vi "AC Transport Measure.vi"(0 "SR860 Ch1 Address":string="4", 1 "Ch1 Enable":bool=TRUE, 2 "Buffer Offset (kb)":string="0", 3 "Buffer Size (kb)":i32=2, 4 "Ch2 Enable":bool, 5 "SR860 Ch2 Address":string="5") -> (12 "R1 Mean":dbl=3.2285320727964972e-06, 13 "R2 Mean":dbl=2.497260236822285e-05, 14 "R1 STD":dbl=8.930686760684023e-10, 15 "T1 Mean":dbl=2.6491355067119002, 16 "T1 STD":dbl=0.013498646334936281, 17 "T2 STD":dbl=2.4806903153139386, 18 "T2 Mean":dbl=-15.289178885519505, 19 "R2 STD":dbl=2.0281499748667416e-06)   [LabVIEW 2020]
uses:
  <vilib>/Analysis/NI_AALBase.lvlib
panel:
  out "Sign2":i8
  out "Garbage 1":string
  out "Sign1":i8
  in  "Sign Correction":bool=TRUE
  out "Garbage Buffer 2":errorcluster
  out "Garbage 2":string
  out "n":i32
  out "number of bytes":i32
  out "cccc":string
  out "#n":string
  out "Garbage Buffer 1":errorcluster
  in  "Measure New?":bool=TRUE
  out "Error SR860 Ch1 2":errorcluster
  out "Buffer 2":sgl[](array[numeric])=[2.0345116e-05, -18.978868, 2.0385167e-05, -18.834179, 2.042573e-05, -18.690664, 2.0466812e-05, -18.548409, 2.0508425e-05, -18.407497, 2.0550568e-05, -18.26797, 2.0593256e-05, -18.129843, 2.0636486e-05, -17.993101, 2.0680263e-05, -17.857708, 2.0724583e-05, -17.723639, 2.0769432e-05, -17.59087, 2.0814796e-05, -17.459414, 2.0860638e-05, -17.32928, 2.0906931e-05, -17.200508, 2.0953643e-05, -17.07314, 2.1000751e-05, -16.947222, 2.1048243e-05, -16.822803, 2.1096113e-05, -16.699953, 2.1144375e-05, -16.578714, 2.1193024e-05, -16.459133, 2.1242071e-05, -16.341232, 2.1291504e-05, -16.224995, 2.134132e-05, -16.110392, 2.1391503e-05, -15.997362, 2.1442036e-05, -15.885857, 2.1492897e-05, -15.775839, 2.1544056e-05, -15.667302, 2.1595477e-05, -15.560262, 2.1647133e-05, -15.454752, 2.1698983e-05, -15.35082, 2.1750997e-05, -15.248506, 2.1803164e-05, -15.147846, 2.1855478e-05, -15.048877, 2.1907945e-05, -14.951616, 2.196056e-05, -14.856077, 2.2013332e-05, -14.762263, 2.2066246e-05, -14.670146, 2.2119291e-05, -14.579687, 2.2172442e-05, -14.490837, 2.2225673e-05, -14.403539, 2.2278957e-05, -14.317757, 2.2332262e-05, -14.233484, 2.238556e-05, -14.150742, 2.243882e-05, -14.069578, 2.2492019e-05, -13.990051, 2.2545135e-05, -13.912204, 2.2598155e-05, -13.836069, 2.2651084e-05, -13.761671, 2.2703925e-05, -13.6890135, 2.2756687e-05, -13.618082, 2.2809376e-05, -13.548866, 2.2861985e-05, -13.481344, 2.2914506e-05, -13.415473, 2.2966908e-05, -13.351213, 2.3019165e-05, -13.288529, 2.307125e-05, -13.22739, 2.312314e-05, -13.167805, 2.317481e-05, -13.109787, 2.3226246e-05, -13.053399, 2.3277438e-05, -12.998701, 2.3328375e-05, -12.945737, 2.3379056e-05, -12.894549, 2.3429491e-05, -12.845147, 2.3479688e-05, -12.797515, 2.3529663e-05, -12.751628, 2.3579429e-05, -12.707447, 2.3628983e-05, -12.664949, 2.3678318e-05, -12.624104, 2.3727416e-05, -12.584871, 2.3776249e-05, -12.547233, 2.3824798e-05, -12.511176, 2.3873035e-05, -12.476706, 2.3920955e-05, -12.44384, 2.3968558e-05, -12.41263, 2.4015842e-05, -12.383121, 2.4062814e-05, -12.355357, 2.4109488e-05, -12.329361, 2.4155874e-05, -12.305133, 2.4201987e-05, -12.282635, 2.4247842e-05, -12.261823, 2.4293442e-05, -12.242645, 2.4338806e-05, -12.225046, 2.4383913e-05, -12.208999, 2.4428757e-05, -12.194475, 2.447331e-05, -12.18147, 2.4517547e-05, -12.169972, 2.456146e-05, -12.159997, 2.4605035e-05, -12.151553, 2.4648285e-05, -12.144676, 2.4691219e-05, -12.139395, 2.4733852e-05, -12.135744, 2.4776204e-05, -12.133726, 2.4818284e-05, -12.133321, 2.4860108e-05, -12.134499, 2.4901683e-05, -12.137181, 2.4943007e-05, -12.141312, 2.4984087e-05, -12.1468315, 2.502491e-05, -12.153699, 2.5065463e-05, -12.161902, 2.5105717e-05, -12.1714325, 2.514566e-05, -12.182309, 2.518527e-05, -12.194537, 2.5224552e-05, -12.20814, 2.5263502e-05, -12.223128, 2.5302144e-05, -12.239519, 2.534049e-05, -12.257316, 2.5378566e-05, -12.276516, 2.5416373e-05, -12.297089, 2.545392e-05, -12.318993, 2.5491205e-05, -12.342162, 2.552821e-05, -12.366525, 2.5564932e-05, -12.392026, 2.5601348e-05, -12.418632, 2.5637439e-05, -12.446331, 2.5673184e-05, -12.475138, 2.570856e-05, -12.505072, 2.574355e-05, -12.536165, 2.577815e-05, -12.568429, 2.5812364e-05, -12.601876, 2.58462e-05, -12.636499, 2.587968e-05, -12.672294, 2.5912816e-05, -12.709234, 2.5945612e-05, -12.747284, 2.5978066e-05, -12.786409, 2.6010159e-05, -12.826544, 2.6041876e-05, -12.867631, 2.607319e-05, -12.90963, 2.6104071e-05, -12.952507, 2.6134505e-05, -12.996262, 2.616447e-05, -13.040911, 2.6193942e-05, -13.086489, 2.622292e-05, -13.133036, 2.6251388e-05, -13.18057, 2.6279351e-05, -13.22909, 2.630681e-05, -13.27858, 2.633379e-05, -13.329011, 2.636029e-05, -13.380347, 2.638632e-05, -13.432542, 2.641187e-05, -13.485546, 2.6436916e-05, -13.539323, 2.6461428e-05, -13.593819, 2.6485382e-05, -13.649003, 2.6508755e-05, -13.704853, 2.6531518e-05, -13.761367, 2.6553664e-05, -13.818572, 2.6575182e-05, -13.876489, 2.6596077e-05, -13.935158, 2.6616346e-05, -13.994596, 2.6635995e-05, -14.054795, 2.6655029e-05, -14.115723, 2.6673462e-05, -14.177329, 2.6691305e-05, -14.239562, 2.6708554e-05, -14.302363, 2.6725202e-05, -14.365683, 2.6741236e-05, -14.429477, 2.6756623e-05, -14.493724, 2.6771333e-05, -14.558396, 2.6785352e-05, -14.62348, 2.6798662e-05, -14.688981, 2.681126e-05, -14.754904, 2.6823154e-05, -14.821272, 2.6834356e-05, -14.888111, 2.6844878e-05, -14.9554205, 2.6854741e-05, -15.023187, 2.6863952e-05, -15.091367, 2.6872523e-05, -15.1599045, 2.6880463e-05, -15.2287245, 2.6887777e-05, -15.297751, 2.6894459e-05, -15.366936, 2.6900496e-05, -15.43625, 2.6905873e-05, -15.505663, 2.6910573e-05, -15.5751705, 2.6914571e-05, -15.644768, 2.6917876e-05, -15.714455, 2.692049e-05, -15.784235, 2.6922431e-05, -15.854111, 2.6923728e-05, -15.924088, 2.6924405e-05, -15.994141, 2.6924477e-05, -16.064253, 2.6923977e-05, -16.134369, 2.6922904e-05, -16.204422, 2.6921272e-05, -16.274336, 2.6919075e-05, -16.34403, 2.691632e-05, -16.413458, 2.6912998e-05, -16.482584, 2.6909103e-05, -16.551395, 2.690463e-05, -16.6199, 2.6899572e-05, -16.688105, 2.6893942e-05, -16.756018, 2.688775e-05, -16.823635, 2.6881024e-05, -16.89094, 2.6873802e-05, -16.957922, 2.6866119e-05, -17.02454, 2.6857995e-05, -17.090763, 2.6849453e-05, -17.156532, 2.6840504e-05, -17.221783, 2.683114e-05, -17.286438, 2.6821364e-05, -17.35044, 2.6811176e-05, -17.413725, 2.6800566e-05, -17.476278, 2.6789536e-05, -17.538095, 2.6778089e-05, -17.599197, 2.6766227e-05, -17.659603, 2.6753964e-05, -17.719322, 2.6741316e-05, -17.77836, 2.6728316e-05, -17.83669, 2.6714988e-05, -17.89429, 2.6701373e-05, -17.951107, 2.6687494e-05, -18.007095, 2.6673364e-05, -18.062208, 2.6658987e-05, -18.116385, 2.6644357e-05, -18.169582, 2.6629465e-05, -18.221745, 2.6614305e-05, -18.27284, 2.6598864e-05, -18.322859, 2.658315e-05, -18.371809, 2.656717e-05, -18.419716, 2.6550935e-05, -18.466608, 2.6534459e-05, -18.512505, 2.6517757e-05, -18.557413, 2.6500858e-05, -18.601297, 2.6483782e-05, -18.644125, 2.646656e-05, -18.685831, 2.64492e-05, -18.726366, 2.6431719e-05, -18.765667, 2.6414105e-05, -18.803701, 2.6396354e-05, -18.84043, 2.6378446e-05, -18.875816, 2.6360369e-05, -18.90985, 2.6342113e-05, -18.942524, 2.6323685e-05, -18.973843, 2.6305092e-05, -19.003841, 2.6286354e-05, -19.032534, 2.6267498e-05, -19.059935, 2.6248541e-05, -19.08605, 2.62295e-05, -19.110842, 2.6210393e-05, -19.13426, 2.6191248e-05, -19.156242, 2.617207e-05, -19.176723, 2.6152864e-05, -19.195648, 2.6133623e-05, -19.212978, 2.6114341e-05, -19.228697, 2.6095006e-05, -19.242796, 2.6075599e-05, -19.255272, 2.6056116e-05, -19.26614, 2.6036569e-05, -19.275402, 2.6016975e-05, -19.28308, 2.5997351e-05, -19.289183, 2.5977739e-05, -19.29372, 2.5958156e-05, -19.296686, 2.5938614e-05, -19.298044, 2.5919142e-05, -19.297743, 2.589974e-05, -19.295721, 2.588042e-05, -19.291908, 2.5861173e-05, -19.286263, 2.5842002e-05, -19.278759]
  out "Buffer 2":string
  out "size(s) 2":i32=512
  out "R2 Buffer":sgl[](array[numeric])=[2.0345116e-05, 2.0385167e-05, 2.042573e-05, 2.0466812e-05, 2.0508425e-05, 2.0550568e-05, 2.0593256e-05, 2.0636486e-05, 2.0680263e-05, 2.0724583e-05, 2.0769432e-05, 2.0814796e-05, 2.0860638e-05, 2.0906931e-05, 2.0953643e-05, 2.1000751e-05, 2.1048243e-05, 2.1096113e-05, 2.1144375e-05, 2.1193024e-05, 2.1242071e-05, 2.1291504e-05, 2.134132e-05, 2.1391503e-05, 2.1442036e-05, 2.1492897e-05, 2.1544056e-05, 2.1595477e-05, 2.1647133e-05, 2.1698983e-05, 2.1750997e-05, 2.1803164e-05, 2.1855478e-05, 2.1907945e-05, 2.196056e-05, 2.2013332e-05, 2.2066246e-05, 2.2119291e-05, 2.2172442e-05, 2.2225673e-05, 2.2278957e-05, 2.2332262e-05, 2.238556e-05, 2.243882e-05, 2.2492019e-05, 2.2545135e-05, 2.2598155e-05, 2.2651084e-05, 2.2703925e-05, 2.2756687e-05, 2.2809376e-05, 2.2861985e-05, 2.2914506e-05, 2.2966908e-05, 2.3019165e-05, 2.307125e-05, 2.312314e-05, 2.317481e-05, 2.3226246e-05, 2.3277438e-05, 2.3328375e-05, 2.3379056e-05, 2.3429491e-05, 2.3479688e-05, 2.3529663e-05, 2.3579429e-05, 2.3628983e-05, 2.3678318e-05, 2.3727416e-05, 2.3776249e-05, 2.3824798e-05, 2.3873035e-05, 2.3920955e-05, 2.3968558e-05, 2.4015842e-05, 2.4062814e-05, 2.4109488e-05, 2.4155874e-05, 2.4201987e-05, 2.4247842e-05, 2.4293442e-05, 2.4338806e-05, 2.4383913e-05, 2.4428757e-05, 2.447331e-05, 2.4517547e-05, 2.456146e-05, 2.4605035e-05, 2.4648285e-05, 2.4691219e-05, 2.4733852e-05, 2.4776204e-05, 2.4818284e-05, 2.4860108e-05, 2.4901683e-05, 2.4943007e-05, 2.4984087e-05, 2.502491e-05, 2.5065463e-05, 2.5105717e-05, 2.514566e-05, 2.518527e-05, 2.5224552e-05, 2.5263502e-05, 2.5302144e-05, 2.534049e-05, 2.5378566e-05, 2.5416373e-05, 2.545392e-05, 2.5491205e-05, 2.552821e-05, 2.5564932e-05, 2.5601348e-05, 2.5637439e-05, 2.5673184e-05, 2.570856e-05, 2.574355e-05, 2.577815e-05, 2.5812364e-05, 2.58462e-05, 2.587968e-05, 2.5912816e-05, 2.5945612e-05, 2.5978066e-05, 2.6010159e-05, 2.6041876e-05, 2.607319e-05, 2.6104071e-05, 2.6134505e-05, 2.616447e-05, 2.6193942e-05, 2.622292e-05, 2.6251388e-05, 2.6279351e-05, 2.630681e-05, 2.633379e-05, 2.636029e-05, 2.638632e-05, 2.641187e-05, 2.6436916e-05, 2.6461428e-05, 2.6485382e-05, 2.6508755e-05, 2.6531518e-05, 2.6553664e-05, 2.6575182e-05, 2.6596077e-05, 2.6616346e-05, 2.6635995e-05, 2.6655029e-05, 2.6673462e-05, 2.6691305e-05, 2.6708554e-05, 2.6725202e-05, 2.6741236e-05, 2.6756623e-05, 2.6771333e-05, 2.6785352e-05, 2.6798662e-05, 2.681126e-05, 2.6823154e-05, 2.6834356e-05, 2.6844878e-05, 2.6854741e-05, 2.6863952e-05, 2.6872523e-05, 2.6880463e-05, 2.6887777e-05, 2.6894459e-05, 2.6900496e-05, 2.6905873e-05, 2.6910573e-05, 2.6914571e-05, 2.6917876e-05, 2.692049e-05, 2.6922431e-05, 2.6923728e-05, 2.6924405e-05, 2.6924477e-05, 2.6923977e-05, 2.6922904e-05, 2.6921272e-05, 2.6919075e-05, 2.691632e-05, 2.6912998e-05, 2.6909103e-05, 2.690463e-05, 2.6899572e-05, 2.6893942e-05, 2.688775e-05, 2.6881024e-05, 2.6873802e-05, 2.6866119e-05, 2.6857995e-05, 2.6849453e-05, 2.6840504e-05, 2.683114e-05, 2.6821364e-05, 2.6811176e-05, 2.6800566e-05, 2.6789536e-05, 2.6778089e-05, 2.6766227e-05, 2.6753964e-05, 2.6741316e-05, 2.6728316e-05, 2.6714988e-05, 2.6701373e-05, 2.6687494e-05, 2.6673364e-05, 2.6658987e-05, 2.6644357e-05, 2.6629465e-05, 2.6614305e-05, 2.6598864e-05, 2.658315e-05, 2.656717e-05, 2.6550935e-05, 2.6534459e-05, 2.6517757e-05, 2.6500858e-05, 2.6483782e-05, 2.646656e-05, 2.64492e-05, 2.6431719e-05, 2.6414105e-05, 2.6396354e-05, 2.6378446e-05, 2.6360369e-05, 2.6342113e-05, 2.6323685e-05, 2.6305092e-05, 2.6286354e-05, 2.6267498e-05, 2.6248541e-05, 2.62295e-05, 2.6210393e-05, 2.6191248e-05, 2.617207e-05, 2.6152864e-05, 2.6133623e-05, 2.6114341e-05, 2.6095006e-05, 2.6075599e-05, 2.6056116e-05, 2.6036569e-05, 2.6016975e-05, 2.5997351e-05, 2.5977739e-05, 2.5958156e-05, 2.5938614e-05, 2.5919142e-05, 2.589974e-05, 2.588042e-05, 2.5861173e-05, 2.5842002e-05]
  out "T2 Buffer":sgl[](array[numeric])=[-18.978868, -18.834179, -18.690664, -18.548409, -18.407497, -18.26797, -18.129843, -17.993101, -17.857708, -17.723639, -17.59087, -17.459414, -17.32928, -17.200508, -17.07314, -16.947222, -16.822803, -16.699953, -16.578714, -16.459133, -16.341232, -16.224995, -16.110392, -15.997362, -15.885857, -15.775839, -15.667302, -15.560262, -15.454752, -15.35082, -15.248506, -15.147846, -15.048877, -14.951616, -14.856077, -14.762263, -14.670146, -14.579687, -14.490837, -14.403539, -14.317757, -14.233484, -14.150742, -14.069578, -13.990051, -13.912204, -13.836069, -13.761671, -13.6890135, -13.618082, -13.548866, -13.481344, -13.415473, -13.351213, -13.288529, -13.22739, -13.167805, -13.109787, -13.053399, -12.998701, -12.945737, -12.894549, -12.845147, -12.797515, -12.751628, -12.707447, -12.664949, -12.624104, -12.584871, -12.547233, -12.511176, -12.476706, -12.44384, -12.41263, -12.383121, -12.355357, -12.329361, -12.305133, -12.282635, -12.261823, -12.242645, -12.225046, -12.208999, -12.194475, -12.18147, -12.169972, -12.159997, -12.151553, -12.144676, -12.139395, -12.135744, -12.133726, -12.133321, -12.134499, -12.137181, -12.141312, -12.1468315, -12.153699, -12.161902, -12.1714325, -12.182309, -12.194537, -12.20814, -12.223128, -12.239519, -12.257316, -12.276516, -12.297089, -12.318993, -12.342162, -12.366525, -12.392026, -12.418632, -12.446331, -12.475138, -12.505072, -12.536165, -12.568429, -12.601876, -12.636499, -12.672294, -12.709234, -12.747284, -12.786409, -12.826544, -12.867631, -12.90963, -12.952507, -12.996262, -13.040911, -13.086489, -13.133036, -13.18057, -13.22909, -13.27858, -13.329011, -13.380347, -13.432542, -13.485546, -13.539323, -13.593819, -13.649003, -13.704853, -13.761367, -13.818572, -13.876489, -13.935158, -13.994596, -14.054795, -14.115723, -14.177329, -14.239562, -14.302363, -14.365683, -14.429477, -14.493724, -14.558396, -14.62348, -14.688981, -14.754904, -14.821272, -14.888111, -14.9554205, -15.023187, -15.091367, -15.1599045, -15.2287245, -15.297751, -15.366936, -15.43625, -15.505663, -15.5751705, -15.644768, -15.714455, -15.784235, -15.854111, -15.924088, -15.994141, -16.064253, -16.134369, -16.204422, -16.274336, -16.34403, -16.413458, -16.482584, -16.551395, -16.6199, -16.688105, -16.756018, -16.823635, -16.89094, -16.957922, -17.02454, -17.090763, -17.156532, -17.221783, -17.286438, -17.35044, -17.413725, -17.476278, -17.538095, -17.599197, -17.659603, -17.719322, -17.77836, -17.83669, -17.89429, -17.951107, -18.007095, -18.062208, -18.116385, -18.169582, -18.221745, -18.27284, -18.322859, -18.371809, -18.419716, -18.466608, -18.512505, -18.557413, -18.601297, -18.644125, -18.685831, -18.726366, -18.765667, -18.803701, -18.84043, -18.875816, -18.90985, -18.942524, -18.973843, -19.003841, -19.032534, -19.059935, -19.08605, -19.110842, -19.13426, -19.156242, -19.176723, -19.195648, -19.212978, -19.228697, -19.242796, -19.255272, -19.26614, -19.275402, -19.28308, -19.289183, -19.29372, -19.296686, -19.298044, -19.297743, -19.295721, -19.291908, -19.286263, -19.278759]
  out "CaptureStat 2":i32=6
  out "T1 Buffer":sgl[](array[numeric])=[2.6467443, 2.6467938, 2.646857, 2.6469476, 2.6470637, 2.6471934, 2.6473505, 2.6475213, 2.6477177, 2.6479414, 2.6481786, 2.6484296, 2.6487062, 2.6489966, 2.6493006, 2.6496317, 2.649963, 2.6503198, 2.6506903, 2.6510746, 2.6514726, 2.6518722, 2.6522956, 2.652707, 2.653146, 2.6535847, 2.6540234, 2.6544743, 2.654927, 2.6553793, 2.6558437, 2.656298, 2.6567504, 2.657203, 2.6576571, 2.6580977, 2.6585383, 2.658979, 2.6593938, 2.6598086, 2.6602237, 2.660613, 2.6610024, 2.661366, 2.6617296, 2.6620662, 2.6623921, 2.662703, 2.66299, 2.663263, 2.6635106, 2.6637464, 2.6639683, 2.664151, 2.6643236, 2.6644688, 2.6646001, 2.664694, 2.6647744, 2.6648169, 2.6648479, 2.6648393, 2.6648307, 2.6647727, 2.664701, 2.6646035, 2.6644824, 2.6643338, 2.6641612, 2.6639752, 2.6637652, 2.6635277, 2.6632802, 2.6630054, 2.6627202, 2.6624076, 2.6620967, 2.6617587, 2.6614106, 2.6610467, 2.6606848, 2.6602988, 2.6599112, 2.65951, 2.6591103, 2.6586971, 2.658284, 2.6578708, 2.6574574, 2.6570306, 2.6566157, 2.6561887, 2.6557739, 2.6553607, 2.654944, 2.654541, 2.654138, 2.6537333, 2.6533542, 2.6529615, 2.6525943, 2.6522274, 2.6518586, 2.6515017, 2.6511567, 2.6508236, 2.6504908, 2.650156, 2.6498349, 2.6495242, 2.6492136, 2.6489146, 2.6486175, 2.6483169, 2.64803, 2.6477416, 2.6474528, 2.6471763, 2.6468878, 2.646611, 2.6463208, 2.6460443, 2.6457658, 2.6454756, 2.6451852, 2.644895, 2.644603, 2.6442993, 2.643997, 2.643693, 2.643377, 2.643049, 2.6427214, 2.6423817, 2.64204, 2.641688, 2.6413364, 2.6409726, 2.640597, 2.6402078, 2.6398203, 2.6394205, 2.6390228, 2.6385994, 2.6381896, 2.6377559, 2.6373222, 2.6368885, 2.6364443, 2.636002, 2.6355479, 2.6350954, 2.6346428, 2.634192, 2.6337295, 2.633282, 2.6328363, 2.6323907, 2.6319468, 2.6315181, 2.631091, 2.630678, 2.63028, 2.629884, 2.6295135, 2.6291463, 2.628805, 2.6284652, 2.6281543, 2.6278691, 2.6275992, 2.6273432, 2.6271162, 2.6269145, 2.6267405, 2.6265798, 2.6264484, 2.6263545, 2.626276, 2.6262383, 2.6262126, 2.626228, 2.6262708, 2.6263528, 2.6264467, 2.6265814, 2.6267557, 2.6269572, 2.6271844, 2.627437, 2.6277308, 2.6280484, 2.6284053, 2.6288013, 2.6292112, 2.6296585, 2.6301434, 2.6306558, 2.631204, 2.6317792, 2.6323924, 2.6330292, 2.6337054, 2.634392, 2.6351295, 2.6358793, 2.6366646, 2.6374638, 2.638297, 2.639144, 2.6400132, 2.6409078, 2.641813, 2.642742, 2.6436691, 2.6446183, 2.6455798, 2.646553, 2.647523, 2.6484911, 2.6494832, 2.6504598, 2.651435, 2.652422, 2.6533918, 2.6543617, 2.655328, 2.6562946, 2.6572456, 2.6581814, 2.6591172, 2.6600375, 2.6609426, 2.661834, 2.6627252, 2.6635876, 2.664436, 2.6652713, 2.6660805, 2.6668866, 2.667667, 2.6684334, 2.6691866, 2.669926, 2.6706517, 2.6713517, 2.6720502, 2.6727228, 2.6733959, 2.674043, 2.6746883, 2.6753201, 2.67594, 2.6765597, 2.677166, 2.6777601]
  out "R1 Buffer":sgl[](array[numeric])=[3.227713e-06, 3.2277464e-06, 3.2277771e-06, 3.227807e-06, 3.2278358e-06, 3.2278624e-06, 3.2278888e-06, 3.2279133e-06, 3.2279372e-06, 3.2279588e-06, 3.2279795e-06, 3.2279997e-06, 3.2280182e-06, 3.2280354e-06, 3.2280523e-06, 3.228067e-06, 3.228082e-06, 3.2280955e-06, 3.228108e-06, 3.2281198e-06, 3.228131e-06, 3.22814e-06, 3.2281503e-06, 3.2281591e-06, 3.2281673e-06, 3.228175e-06, 3.2281823e-06, 3.2281896e-06, 3.2281955e-06, 3.2282019e-06, 3.228208e-06, 3.2282135e-06, 3.2282192e-06, 3.2282244e-06, 3.2282292e-06, 3.2282346e-06, 3.2282394e-06, 3.228245e-06, 3.2282503e-06, 3.2282558e-06, 3.228261e-06, 3.2282665e-06, 3.2282721e-06, 3.2282787e-06, 3.2282844e-06, 3.2282906e-06, 3.2282971e-06, 3.2283046e-06, 3.2283117e-06, 3.228319e-06, 3.228327e-06, 3.2283347e-06, 3.2283433e-06, 3.2283515e-06, 3.2283597e-06, 3.2283688e-06, 3.2283783e-06, 3.2283872e-06, 3.2283976e-06, 3.2284067e-06, 3.2284163e-06, 3.2284265e-06, 3.2284363e-06, 3.228446e-06, 3.228456e-06, 3.2284656e-06, 3.2284747e-06, 3.2284845e-06, 3.228494e-06, 3.2285034e-06, 3.2285122e-06, 3.2285218e-06, 3.2285302e-06, 3.2285388e-06, 3.2285468e-06, 3.2285552e-06, 3.228563e-06, 3.2285714e-06, 3.228579e-06, 3.2285868e-06, 3.2285943e-06, 3.2286023e-06, 3.2286098e-06, 3.2286177e-06, 3.2286255e-06, 3.228633e-06, 3.2286412e-06, 3.2286493e-06, 3.2286578e-06, 3.2286666e-06, 3.2286757e-06, 3.2286846e-06, 3.2286948e-06, 3.2287046e-06, 3.2287155e-06, 3.2287267e-06, 3.2287376e-06, 3.22875e-06, 3.228764e-06, 3.228777e-06, 3.228791e-06, 3.2288065e-06, 3.2288224e-06, 3.228839e-06, 3.2288556e-06, 3.2288744e-06, 3.228893e-06, 3.2289136e-06, 3.228934e-06, 3.2289554e-06, 3.228978e-06, 3.229001e-06, 3.2290245e-06, 3.2290488e-06, 3.2290739e-06, 3.2290998e-06, 3.2291262e-06, 3.2291534e-06, 3.2291807e-06, 3.229209e-06, 3.2292362e-06, 3.2292648e-06, 3.2292937e-06, 3.229323e-06, 3.229352e-06, 3.2293808e-06, 3.2294106e-06, 3.2294395e-06, 3.2294686e-06, 3.2294981e-06, 3.2295268e-06, 3.2295554e-06, 3.2295834e-06, 3.2296114e-06, 3.2296396e-06, 3.2296655e-06, 3.2296923e-06, 3.2297182e-06, 3.2297426e-06, 3.229767e-06, 3.2297908e-06, 3.2298135e-06, 3.2298346e-06, 3.2298558e-06, 3.2298756e-06, 3.2298938e-06, 3.2299113e-06, 3.2299274e-06, 3.2299426e-06, 3.2299554e-06, 3.2299686e-06, 3.2299783e-06, 3.2299881e-06, 3.2299956e-06, 3.2300009e-06, 3.2300045e-06, 3.230007e-06, 3.2300072e-06, 3.2300063e-06, 3.2300018e-06, 3.2299965e-06, 3.229989e-06, 3.2299795e-06, 3.229967e-06, 3.2299529e-06, 3.2299372e-06, 3.2299192e-06, 3.229899e-06, 3.2298758e-06, 3.2298508e-06, 3.2298242e-06, 3.2297953e-06, 3.2297637e-06, 3.2297294e-06, 3.229694e-06, 3.2296562e-06, 3.2296157e-06, 3.229574e-06, 3.2295304e-06, 3.2294834e-06, 3.2294358e-06, 3.229386e-06, 3.2293347e-06, 3.2292812e-06, 3.2292264e-06, 3.22917e-06, 3.229112e-06, 3.229053e-06, 3.2289927e-06, 3.2289308e-06, 3.2288679e-06, 3.2288053e-06, 3.228741e-06, 3.228675e-06, 3.2286107e-06, 3.2285445e-06, 3.2284781e-06, 3.2284122e-06, 3.2283467e-06, 3.2282799e-06, 3.2282148e-06, 3.2281503e-06, 3.2280855e-06, 3.228022e-06, 3.2279593e-06, 3.227898e-06, 3.2278379e-06, 3.2277792e-06, 3.227722e-06, 3.2276666e-06, 3.2276134e-06, 3.2275611e-06, 3.2275123e-06, 3.2274643e-06, 3.2274188e-06, 3.2273763e-06, 3.2273354e-06, 3.2272965e-06, 3.2272612e-06, 3.2272276e-06, 3.2271962e-06, 3.227167e-06, 3.2271405e-06, 3.2271166e-06, 3.2270955e-06, 3.227076e-06, 3.227059e-06, 3.2270439e-06, 3.2270318e-06, 3.2270211e-06, 3.2270136e-06, 3.2270077e-06, 3.2270038e-06, 3.2270013e-06, 3.2270013e-06, 3.2270032e-06, 3.2270068e-06, 3.2270118e-06, 3.2270184e-06, 3.2270261e-06, 3.2270352e-06, 3.2270457e-06, 3.227058e-06, 3.2270711e-06, 3.2270848e-06, 3.2270993e-06, 3.2271155e-06, 3.2271316e-06, 3.2271491e-06, 3.2271666e-06, 3.2271848e-06, 3.2272035e-06, 3.2272226e-06, 3.2272421e-06, 3.2272621e-06, 3.2272826e-06]
  out "Error SR860 Ch1":errorcluster
  out "Buffer 1":sgl[](array[numeric])=[3.227713e-06, 2.6467443, 3.2277464e-06, 2.6467938, 3.2277771e-06, 2.646857, 3.227807e-06, 2.6469476, 3.2278358e-06, 2.6470637, 3.2278624e-06, 2.6471934, 3.2278888e-06, 2.6473505, 3.2279133e-06, 2.6475213, 3.2279372e-06, 2.6477177, 3.2279588e-06, 2.6479414, 3.2279795e-06, 2.6481786, 3.2279997e-06, 2.6484296, 3.2280182e-06, 2.6487062, 3.2280354e-06, 2.6489966, 3.2280523e-06, 2.6493006, 3.228067e-06, 2.6496317, 3.228082e-06, 2.649963, 3.2280955e-06, 2.6503198, 3.228108e-06, 2.6506903, 3.2281198e-06, 2.6510746, 3.228131e-06, 2.6514726, 3.22814e-06, 2.6518722, 3.2281503e-06, 2.6522956, 3.2281591e-06, 2.652707, 3.2281673e-06, 2.653146, 3.228175e-06, 2.6535847, 3.2281823e-06, 2.6540234, 3.2281896e-06, 2.6544743, 3.2281955e-06, 2.654927, 3.2282019e-06, 2.6553793, 3.228208e-06, 2.6558437, 3.2282135e-06, 2.656298, 3.2282192e-06, 2.6567504, 3.2282244e-06, 2.657203, 3.2282292e-06, 2.6576571, 3.2282346e-06, 2.6580977, 3.2282394e-06, 2.6585383, 3.228245e-06, 2.658979, 3.2282503e-06, 2.6593938, 3.2282558e-06, 2.6598086, 3.228261e-06, 2.6602237, 3.2282665e-06, 2.660613, 3.2282721e-06, 2.6610024, 3.2282787e-06, 2.661366, 3.2282844e-06, 2.6617296, 3.2282906e-06, 2.6620662, 3.2282971e-06, 2.6623921, 3.2283046e-06, 2.662703, 3.2283117e-06, 2.66299, 3.228319e-06, 2.663263, 3.228327e-06, 2.6635106, 3.2283347e-06, 2.6637464, 3.2283433e-06, 2.6639683, 3.2283515e-06, 2.664151, 3.2283597e-06, 2.6643236, 3.2283688e-06, 2.6644688, 3.2283783e-06, 2.6646001, 3.2283872e-06, 2.664694, 3.2283976e-06, 2.6647744, 3.2284067e-06, 2.6648169, 3.2284163e-06, 2.6648479, 3.2284265e-06, 2.6648393, 3.2284363e-06, 2.6648307, 3.228446e-06, 2.6647727, 3.228456e-06, 2.664701, 3.2284656e-06, 2.6646035, 3.2284747e-06, 2.6644824, 3.2284845e-06, 2.6643338, 3.228494e-06, 2.6641612, 3.2285034e-06, 2.6639752, 3.2285122e-06, 2.6637652, 3.2285218e-06, 2.6635277, 3.2285302e-06, 2.6632802, 3.2285388e-06, 2.6630054, 3.2285468e-06, 2.6627202, 3.2285552e-06, 2.6624076, 3.228563e-06, 2.6620967, 3.2285714e-06, 2.6617587, 3.228579e-06, 2.6614106, 3.2285868e-06, 2.6610467, 3.2285943e-06, 2.6606848, 3.2286023e-06, 2.6602988, 3.2286098e-06, 2.6599112, 3.2286177e-06, 2.65951, 3.2286255e-06, 2.6591103, 3.228633e-06, 2.6586971, 3.2286412e-06, 2.658284, 3.2286493e-06, 2.6578708, 3.2286578e-06, 2.6574574, 3.2286666e-06, 2.6570306, 3.2286757e-06, 2.6566157, 3.2286846e-06, 2.6561887, 3.2286948e-06, 2.6557739, 3.2287046e-06, 2.6553607, 3.2287155e-06, 2.654944, 3.2287267e-06, 2.654541, 3.2287376e-06, 2.654138, 3.22875e-06, 2.6537333, 3.228764e-06, 2.6533542, 3.228777e-06, 2.6529615, 3.228791e-06, 2.6525943, 3.2288065e-06, 2.6522274, 3.2288224e-06, 2.6518586, 3.228839e-06, 2.6515017, 3.2288556e-06, 2.6511567, 3.2288744e-06, 2.6508236, 3.228893e-06, 2.6504908, 3.2289136e-06, 2.650156, 3.228934e-06, 2.6498349, 3.2289554e-06, 2.6495242, 3.228978e-06, 2.6492136, 3.229001e-06, 2.6489146, 3.2290245e-06, 2.6486175, 3.2290488e-06, 2.6483169, 3.2290739e-06, 2.64803, 3.2290998e-06, 2.6477416, 3.2291262e-06, 2.6474528, 3.2291534e-06, 2.6471763, 3.2291807e-06, 2.6468878, 3.229209e-06, 2.646611, 3.2292362e-06, 2.6463208, 3.2292648e-06, 2.6460443, 3.2292937e-06, 2.6457658, 3.229323e-06, 2.6454756, 3.229352e-06, 2.6451852, 3.2293808e-06, 2.644895, 3.2294106e-06, 2.644603, 3.2294395e-06, 2.6442993, 3.2294686e-06, 2.643997, 3.2294981e-06, 2.643693, 3.2295268e-06, 2.643377, 3.2295554e-06, 2.643049, 3.2295834e-06, 2.6427214, 3.2296114e-06, 2.6423817, 3.2296396e-06, 2.64204, 3.2296655e-06, 2.641688, 3.2296923e-06, 2.6413364, 3.2297182e-06, 2.6409726, 3.2297426e-06, 2.640597, 3.229767e-06, 2.6402078, 3.2297908e-06, 2.6398203, 3.2298135e-06, 2.6394205, 3.2298346e-06, 2.6390228, 3.2298558e-06, 2.6385994, 3.2298756e-06, 2.6381896, 3.2298938e-06, 2.6377559, 3.2299113e-06, 2.6373222, 3.2299274e-06, 2.6368885, 3.2299426e-06, 2.6364443, 3.2299554e-06, 2.636002, 3.2299686e-06, 2.6355479, 3.2299783e-06, 2.6350954, 3.2299881e-06, 2.6346428, 3.2299956e-06, 2.634192, 3.2300009e-06, 2.6337295, 3.2300045e-06, 2.633282, 3.230007e-06, 2.6328363, 3.2300072e-06, 2.6323907, 3.2300063e-06, 2.6319468, 3.2300018e-06, 2.6315181, 3.2299965e-06, 2.631091, 3.229989e-06, 2.630678, 3.2299795e-06, 2.63028, 3.229967e-06, 2.629884, 3.2299529e-06, 2.6295135, 3.2299372e-06, 2.6291463, 3.2299192e-06, 2.628805, 3.229899e-06, 2.6284652, 3.2298758e-06, 2.6281543, 3.2298508e-06, 2.6278691, 3.2298242e-06, 2.6275992, 3.2297953e-06, 2.6273432, 3.2297637e-06, 2.6271162, 3.2297294e-06, 2.6269145, 3.229694e-06, 2.6267405, 3.2296562e-06, 2.6265798, 3.2296157e-06, 2.6264484, 3.229574e-06, 2.6263545, 3.2295304e-06, 2.626276, 3.2294834e-06, 2.6262383, 3.2294358e-06, 2.6262126, 3.229386e-06, 2.626228, 3.2293347e-06, 2.6262708, 3.2292812e-06, 2.6263528, 3.2292264e-06, 2.6264467, 3.22917e-06, 2.6265814, 3.229112e-06, 2.6267557, 3.229053e-06, 2.6269572, 3.2289927e-06, 2.6271844, 3.2289308e-06, 2.627437, 3.2288679e-06, 2.6277308, 3.2288053e-06, 2.6280484, 3.228741e-06, 2.6284053, 3.228675e-06, 2.6288013, 3.2286107e-06, 2.6292112, 3.2285445e-06, 2.6296585, 3.2284781e-06, 2.6301434, 3.2284122e-06, 2.6306558, 3.2283467e-06, 2.631204, 3.2282799e-06, 2.6317792, 3.2282148e-06, 2.6323924, 3.2281503e-06, 2.6330292, 3.2280855e-06, 2.6337054, 3.228022e-06, 2.634392, 3.2279593e-06, 2.6351295, 3.227898e-06, 2.6358793, 3.2278379e-06, 2.6366646, 3.2277792e-06, 2.6374638, 3.227722e-06, 2.638297, 3.2276666e-06, 2.639144, 3.2276134e-06, 2.6400132, 3.2275611e-06, 2.6409078, 3.2275123e-06, 2.641813, 3.2274643e-06, 2.642742, 3.2274188e-06, 2.6436691, 3.2273763e-06, 2.6446183, 3.2273354e-06, 2.6455798, 3.2272965e-06, 2.646553, 3.2272612e-06, 2.647523, 3.2272276e-06, 2.6484911, 3.2271962e-06, 2.6494832, 3.227167e-06, 2.6504598, 3.2271405e-06, 2.651435, 3.2271166e-06, 2.652422, 3.2270955e-06, 2.6533918, 3.227076e-06, 2.6543617, 3.227059e-06, 2.655328, 3.2270439e-06, 2.6562946, 3.2270318e-06, 2.6572456, 3.2270211e-06, 2.6581814, 3.2270136e-06, 2.6591172, 3.2270077e-06, 2.6600375, 3.2270038e-06, 2.6609426, 3.2270013e-06, 2.661834, 3.2270013e-06, 2.6627252, 3.2270032e-06, 2.6635876, 3.2270068e-06, 2.664436, 3.2270118e-06, 2.6652713, 3.2270184e-06, 2.6660805, 3.2270261e-06, 2.6668866, 3.2270352e-06, 2.667667, 3.2270457e-06, 2.6684334, 3.227058e-06, 2.6691866, 3.2270711e-06, 2.669926, 3.2270848e-06, 2.6706517, 3.2270993e-06, 2.6713517, 3.2271155e-06, 2.6720502, 3.2271316e-06, 2.6727228, 3.2271491e-06, 2.6733959, 3.2271666e-06, 2.674043, 3.2271848e-06, 2.6746883, 3.2272035e-06, 2.6753201, 3.2272226e-06, 2.67594, 3.2272421e-06, 2.6765597, 3.2272621e-06, 2.677166, 3.2272826e-06, 2.6777601]
  out "Buffer 1":string
  out "size(s) 1":i32=512
  out "CaptureStat 1":i32=6
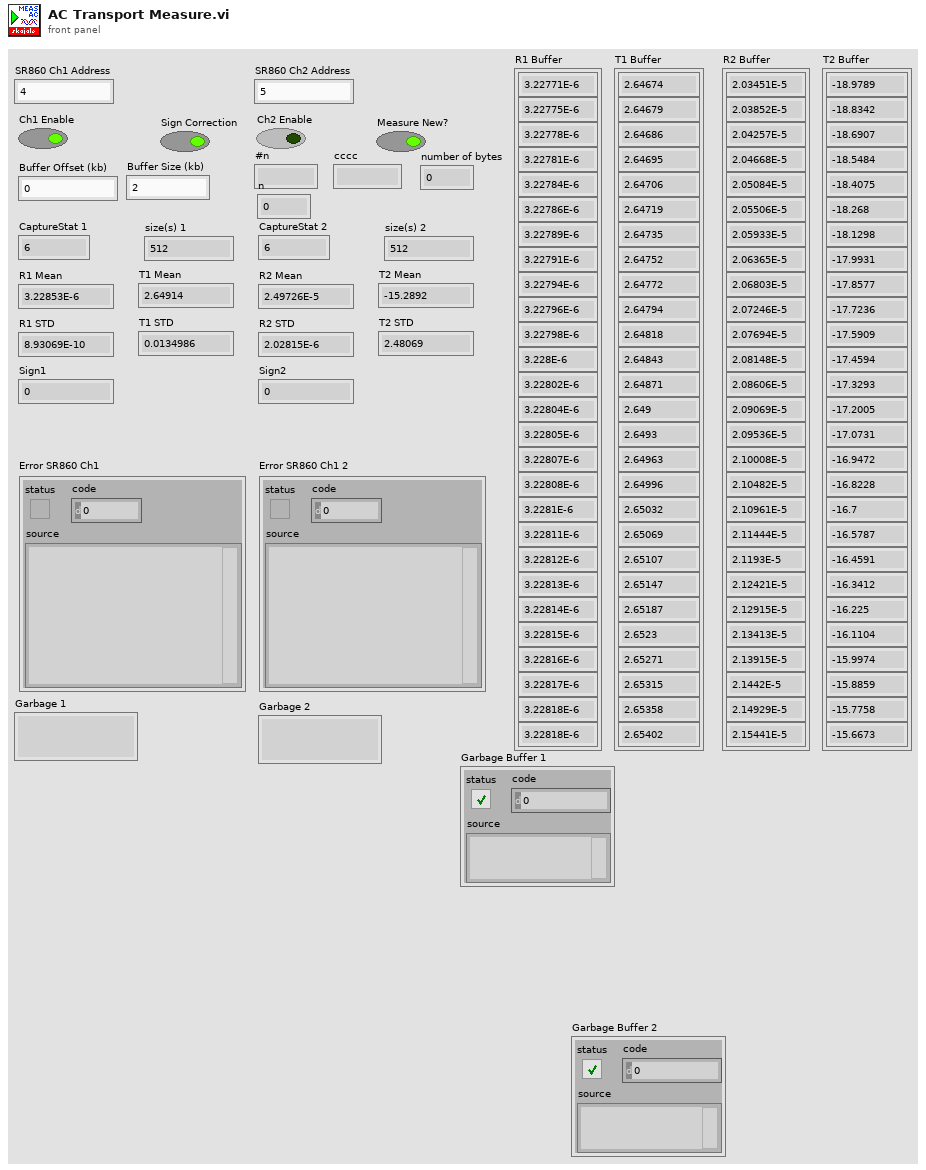
[diagram p1: front panel]
types:
  T1 = enum16{"big-endian, network order", "native, host order", "little-endian"}
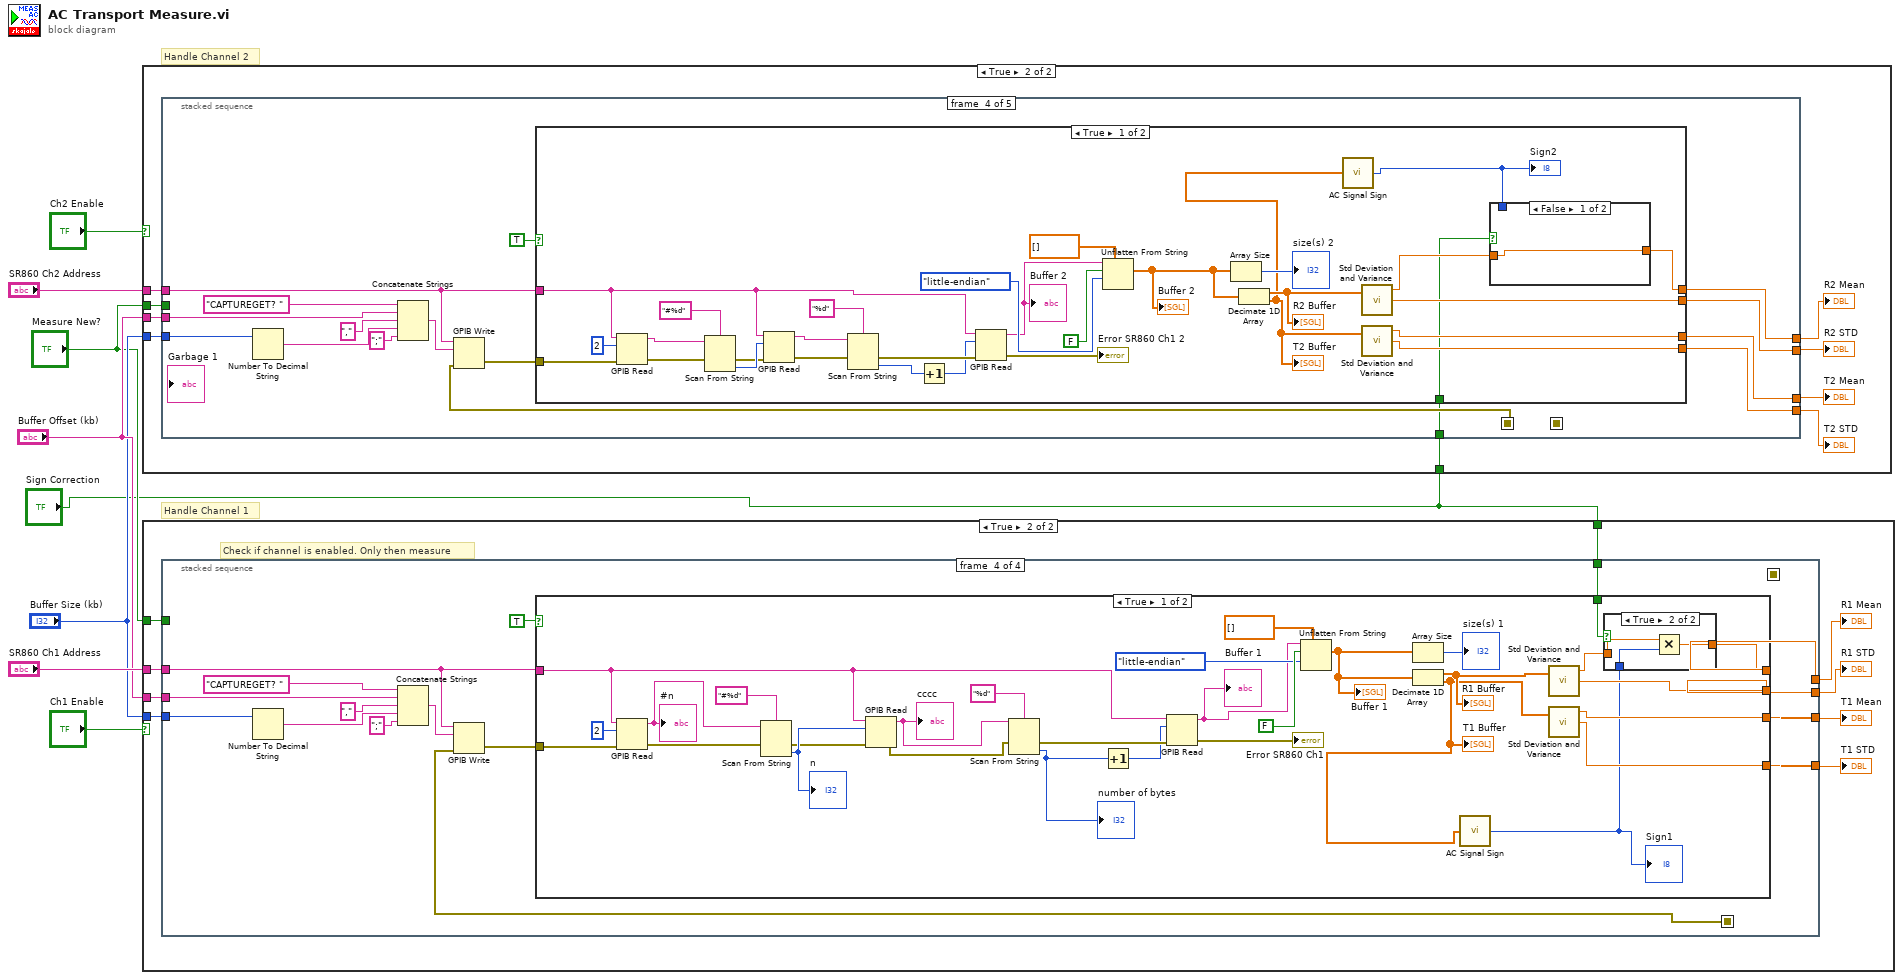
[diagram p0: block diagram]
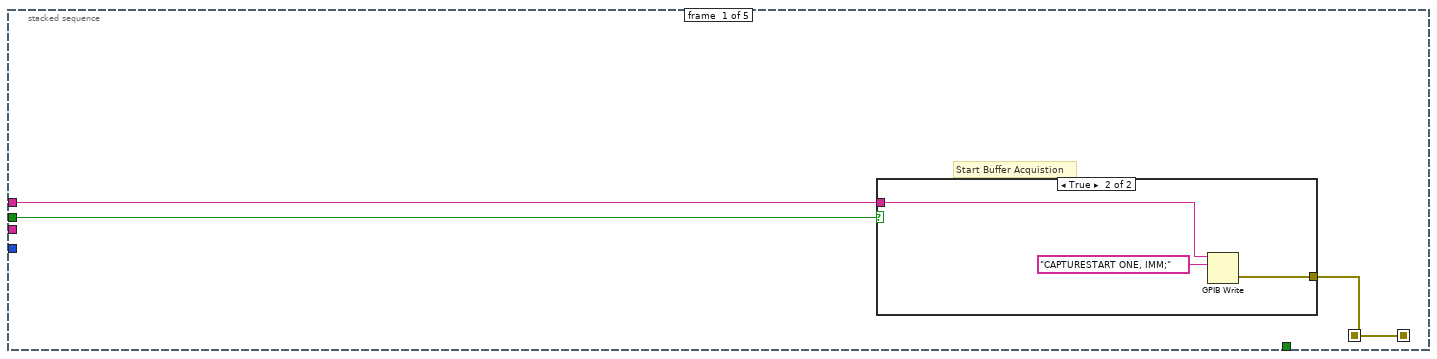
[diagram p3: hidden frame]
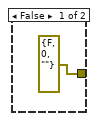
[diagram p4: hidden frame]
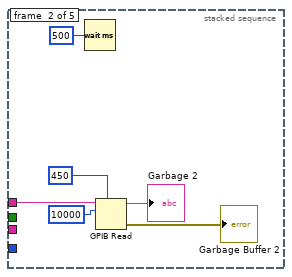
[diagram p5: hidden frame]
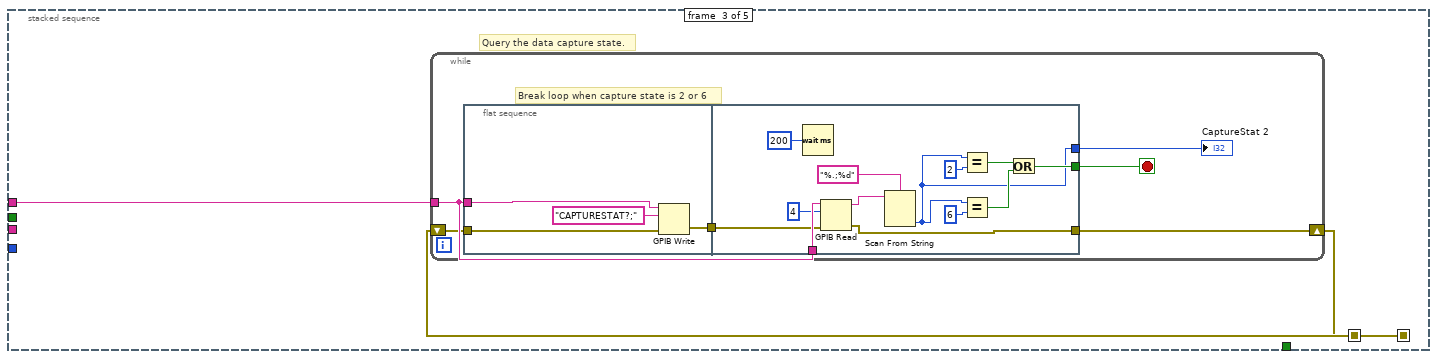
[diagram p6: hidden frame]
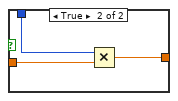
[diagram p7: hidden frame]
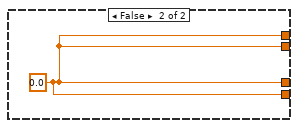
[diagram p8: hidden frame]
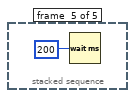
[diagram p9: hidden frame]
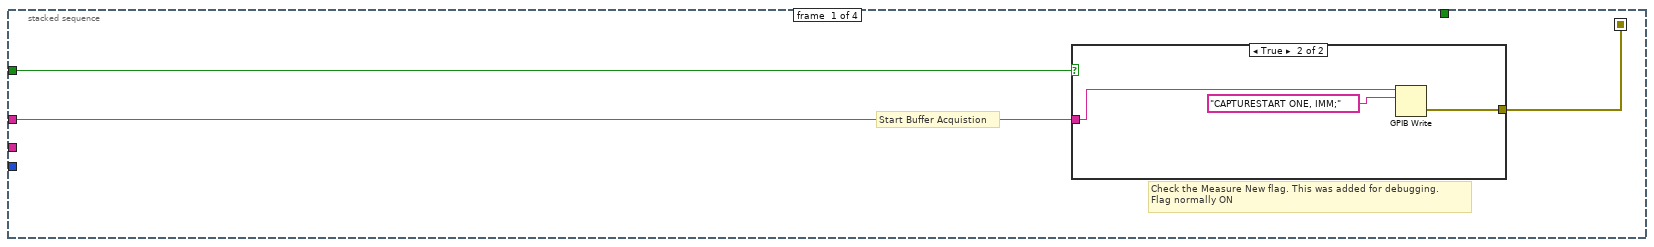
[diagram p11: hidden frame]
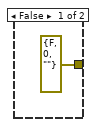
[diagram p12: hidden frame]
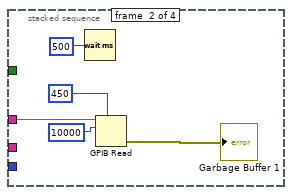
[diagram p13: hidden frame]
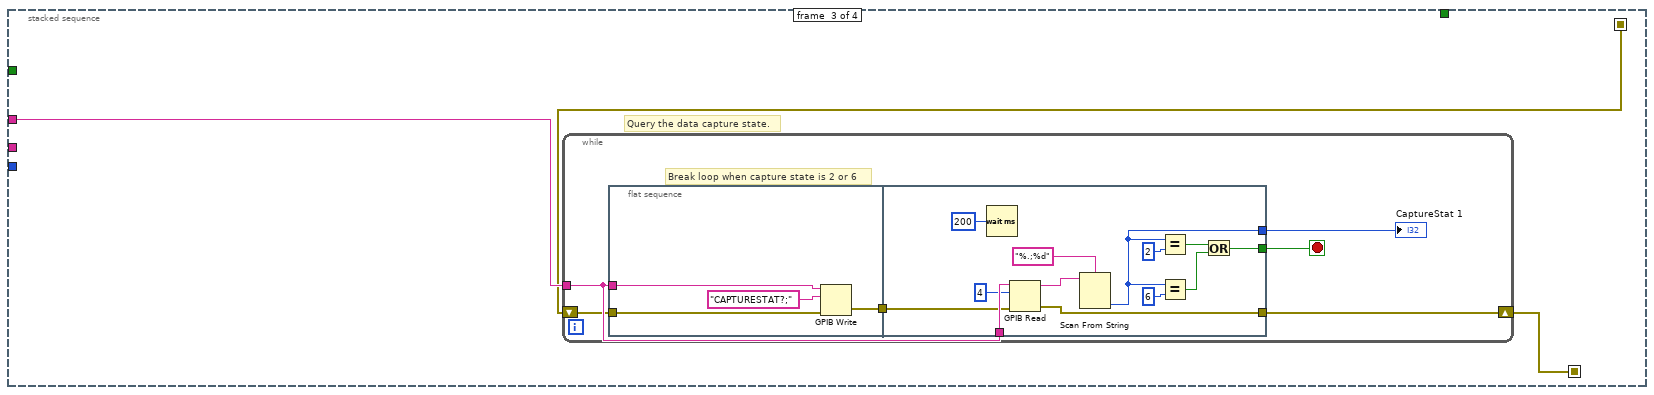
[diagram p14: hidden frame]
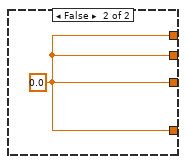
[diagram p16: hidden frame]
diagram:
  # "Handle Channel 2"
  # "Handle Channel 1"
  n1 = case shown="True" "Ch2 Enable" {
    tunnel: "SR860 Ch2 Address" -> [_ w17]
    tunnel: "Buffer Offset (kb)" -> [_ w12]
    tunnel: "Buffer Size (kb)" -> [_ w11]
    tunnel: "Measure New?" -> [_ w10]
    tunnel: "Sign Correction" -> [_ w9]
    frame False {
    }
    frame True {
      n2 = stacked-sequence {
        seq-local: [w19 _ _ _ _] -> [_ _ w32 _ _]
        seq-local: [_ _ w31 _ _] -> [_ _ _ w65 _]
        tunnel: w17 -> [w20 w26 w33 w68 _]
        tunnel: [_ _ _ w63 _] -> w13
        tunnel: [_ _ _ w62 _] -> w14
        tunnel: [_ _ _ w61 _] -> w15
        tunnel: [_ _ _ w60 _] -> w16
        tunnel: w12 -> [_ _ _ w59 _]
        tunnel: w11 -> [_ _ _ w58 _]
        tunnel: w10 -> [w18 _ _ _ _]
        tunnel: w9 -> [_ _ _ w57 _]
        frame #0 {
          # "Start Buffer Acquistion"
          n3 = case shown="True" w18 {
            tunnel: w20 -> [_ w23]
            tunnel: [errorcluster {"status"=FALSE, "code"=0, "source"=""} ("error out") w22] -> w19
            frame False {
            }
            frame True {
              n4 = GPIB Write(0:w23, 1:"CAPTURESTART ONE, IMM;" ("data")) -> (6:w22:errorcluster)  [unwired: 3 in, 1 out]
            }
          }
        }
        frame #1 {
          n5 = Wait (ms)(milliseconds to wait=u32 500) -> ()  [unwired: 1 out]
          n6 = GPIB Read(0:w26, 1:10000 ("byte count"), 4:450 ("timeout ms (488.2 global)")) -> (5:→"Garbage 2":string, 7:→"Garbage Buffer 2":errorcluster)  [unwired: 2 in, 1 out]
        }
        frame #2 {
          # "Query the data capture state."
          n7 = while {
            tunnel: w33 -> [w38]
            shift-right: [w34] -> w31
            shift-left: w32 -> [w35]
            stop <- w37 stop-if-true
            # "Break loop when capture state is 2 or 6"
            n8 = flat-sequence {
              tunnel: w38 -> [w41]
              tunnel: [w42] -> w39
              tunnel: w35 -> [w40]
              tunnel: w39 -> [w49]
              tunnel: w38 -> [w51]
              tunnel: [w47] -> w37
              tunnel: [w46] -> w36
              tunnel: [w44] -> w34
              frame #0 {
                n9 = GPIB Write(0:w41, 1:"CAPTURESTAT?;", 3:w40) -> (6:w42:errorcluster)  [unwired: 2 in, 1 out]
              }
              frame #1 {
                n10 = Wait (ms)(milliseconds to wait=u32 200) -> ()  [unwired: 1 out]
                n11 = GPIB Read(0:w51, 1:u32 4 ("byte count"), 3:w49) -> (5:w54:string, 7:w44:errorcluster)  [unwired: 2 in, 1 out]
                n12 = Scan From String(format string="%.;%d", input string=w54) -> (output 1=w46:i32)  [unwired: 3 in, 3 out]
                n13 = Equal?(x=w46, y=2) -> (x = y?=w55:bool)
                n14 = Equal?(x=w46, y=6) -> (x = y?=w56:bool)
                n15 = Or(x=w55, y=w56) -> (x .or. y?=w47:bool)
              }
            }
            "CaptureStat 2" <- w36
          }
        }
        frame #3 {
          n16 = Number To Decimal String(number=w58) -> (decimal integer string=w64:string)  [unwired: 1 in]
          n17 = Concatenate Strings("CAPTUREGET? " ("data"), w59, "," ("string"), w64, ";" ("string")) -> (w69:string)
          n18 = GPIB Write(0:w68, 1:w69, 3:w65) -> (6:w66:errorcluster)  [unwired: 2 in, 1 out]
          n19 = case shown="True" TRUE {
            tunnel: w68 -> [w82 _]
            tunnel: w66 -> [w86 _]
            tunnel: [w83 w107] -> w63
            tunnel: [w79 w107] -> w62
            tunnel: [w78 w107] -> w61
            tunnel: [w76 w107] -> w60
            tunnel: w57 -> [w75 _]
            frame True {
              n20 = GPIB Read(0:w82, 1:u32 2 ("byte count"), 3:w86) -> (5:w91:string, 7:w95:errorcluster)  [unwired: 2 in, 1 out]
              n21 = Scan From String(format string="#%d", input string=w91, error in=w95) -> (error out=w99:errorcluster, output 1=w101:i32)  [unwired: 1 in, 3 out]
              n22 = GPIB Read(0:w82, 1:w101, 3:w99) -> (5:w90:string, 7:w98:errorcluster)  [unwired: 2 in, 1 out]
              n23 = Scan From String(format string="%d", input string=w90, error in=w98) -> (error out=w97:errorcluster, output 1=w80:i32)  [unwired: 1 in, 3 out]
              n24 = Increment(x=w80) -> (x+1=w81:i32)
              n25 = GPIB Read(0:w82, 1:w81, 3:w97) -> (5:w89:string, 7:→"Error SR860 Ch1 2":errorcluster)  [unwired: 2 in, 1 out]
              "Buffer 2" <- w89
              n26 = Unflatten From String(type=sgl[] [], binary string=w89, data includes array or string size? (T)=FALSE, byte order (0:big-endian, network order)=T1."little-endian") -> (value=w85:sgl[])  [unwired: 1 in, 2 out]
              "Buffer 2" <- w85
              n27 = Array Size(array=w85) -> (size(s)=→"size(s) 2":i32)
              n28 = Decimate 1D Array(w85) -> (w84:sgl[], w74:sgl[])
              "R2 Buffer" <- w84
              "T2 Buffer" <- w74
              n29 = call "AC Signal Sign.vi"("Array"=w74) -> ("Sign1"=w73:i8)
              "Sign2" <- w73
              n30 = call <vilib>:"Std Deviation and Variance.vi"("X"=w84) -> ("mean"=w77:dbl, "standard deviation"=w78:dbl)  [unwired: 1 in, 1 out]
              n31 = call <vilib>:"Std Deviation and Variance.vi"("X"=w74) -> ("mean"=w79:dbl, "standard deviation"=w83:dbl)  [unwired: 1 in, 1 out]
              n32 = case shown="False" w75 {
                tunnel: w73 -> [_ w106]
                tunnel: w77 -> [w103 w105]
                tunnel: [w103 w104] -> w76
                frame False {
                }
                frame True {
                  n33 = Multiply(x=w106, y=w105) -> (x*y=w104:dbl)
                }
              }
            }
            frame False {
              w107 = 0.0
            }
          }
        }
        frame #4 {
          n34 = Wait (ms)(milliseconds to wait=u32 200) -> ()  [unwired: 1 out]
        }
      }
      "R2 Mean" <- w16
      "R2 STD" <- w15
      "T2 Mean" <- w14
      "T2 STD" <- w13
    }
  }
  n35 = case shown="True" "Ch1 Enable" {
    tunnel: "SR860 Ch1 Address" -> [_ w117]
    tunnel: "Buffer Offset (kb)" -> [_ w112]
    tunnel: "Buffer Size (kb)" -> [_ w111]
    tunnel: "Measure New?" -> [_ w110]
    tunnel: "Sign Correction" -> [_ w109]
    frame False {
    }
    frame True {
      # "Check if channel is enabled. Only then measure"
      n36 = stacked-sequence {
        seq-local: [w119 _ _ _] -> [_ _ w131 _]
        seq-local: [_ _ w130 _] -> [_ _ _ w164]
        tunnel: w117 -> [w120 w128 w132 w167]
        tunnel: [_ _ _ w162] -> w113
        tunnel: [_ _ _ w161] -> w114
        tunnel: [_ _ _ w160] -> w115
        tunnel: [_ _ _ w157] -> w116
        tunnel: w112 -> [_ _ _ w159]
        tunnel: w111 -> [_ _ _ w158]
        tunnel: w110 -> [w118 _ _ _]
        tunnel: w109 -> [_ _ _ w156]
        frame #0 {
          # "Check the Measure New flag. This was added for debugging.\nFlag normally ON"
          # "Start Buffer Acquistion"
          n37 = case shown="True" w118 {
            tunnel: w120 -> [_ w123]
            tunnel: [errorcluster {"status"=FALSE, "code"=0, "source"=""} ("error out") w122] -> w119
            frame False {
            }
            frame True {
              n38 = GPIB Write(0:w123, 1:"CAPTURESTART ONE, IMM;" ("data")) -> (6:w122:errorcluster)  [unwired: 3 in, 1 out]
            }
          }
        }
        frame #1 {
          n39 = Wait (ms)(milliseconds to wait=u32 500) -> ()  [unwired: 1 out]
          n40 = GPIB Read(0:w128, 1:10000 ("byte count"), 4:450 ("timeout ms (488.2 global)")) -> (7:→"Garbage Buffer 1":errorcluster)  [unwired: 2 in, 2 out]
        }
        frame #2 {
          # "Query the data capture state."
          n41 = while {
            tunnel: w132 -> [w137]
            shift-right: [w133] -> w130
            shift-left: w131 -> [w134]
            stop <- w136 stop-if-true
            # "Break loop when capture state is 2 or 6"
            n42 = flat-sequence {
              tunnel: w137 -> [w140]
              tunnel: [w141] -> w138
              tunnel: w134 -> [w139]
              tunnel: w138 -> [w148]
              tunnel: w137 -> [w150]
              tunnel: [w146] -> w136
              tunnel: [w145] -> w135
              tunnel: [w143] -> w133
              frame #0 {
                n43 = GPIB Write(0:w140, 1:"CAPTURESTAT?;", 3:w139) -> (6:w141:errorcluster)  [unwired: 2 in, 1 out]
              }
              frame #1 {
                n44 = Wait (ms)(milliseconds to wait=u32 200) -> ()  [unwired: 1 out]
                n45 = GPIB Read(0:w150, 1:u32 4 ("byte count"), 3:w148) -> (5:w153:string, 7:w143:errorcluster)  [unwired: 2 in, 1 out]
                n46 = Scan From String(format string="%.;%d", input string=w153) -> (output 1=w145:i32)  [unwired: 3 in, 3 out]
                n47 = Equal?(x=w145, y=2) -> (x = y?=w154:bool)
                n48 = Equal?(x=w145, y=6) -> (x = y?=w155:bool)
                n49 = Or(x=w154, y=w155) -> (x .or. y?=w146:bool)
              }
            }
            "CaptureStat 1" <- w135
          }
        }
        frame #3 {
          n50 = Number To Decimal String(number=w158) -> (decimal integer string=w163:string)  [unwired: 1 in]
          n51 = Concatenate Strings("CAPTUREGET? " ("data"), w159, "," ("string"), w163, ";" ("string")) -> (w168:string)
          n52 = GPIB Write(0:w167, 1:w168, 3:w164) -> (6:w165:errorcluster)  [unwired: 2 in, 1 out]
          n53 = case shown="True" TRUE {
            tunnel: w167 -> [w181 _]
            tunnel: w165 -> [w185 _]
            tunnel: [w182 w206] -> w162
            tunnel: [w178 w206] -> w161
            tunnel: [w177 w206] -> w160
            tunnel: [w175 w206] -> w157
            tunnel: w156 -> [w174 _]
            frame True {
              n54 = GPIB Read(0:w181, 1:u32 2 ("byte count"), 3:w185) -> (5:w190:string, 7:w194:errorcluster)  [unwired: 2 in, 1 out]
              "#n" <- w190
              n55 = Scan From String(format string="#%d", input string=w190, error in=w194) -> (error out=w198:errorcluster, output 1=w200:i32)  [unwired: 1 in, 3 out]
              "n" <- w200
              n56 = GPIB Read(0:w181, 1:w200, 3:w198) -> (5:w189:string, 7:w197:errorcluster)  [unwired: 2 in, 1 out]
              "cccc" <- w189
              n57 = Scan From String(format string="%d", input string=w189, error in=w197) -> (error out=w196:errorcluster, output 1=w179:i32)  [unwired: 1 in, 3 out]
              "number of bytes" <- w179
              n58 = Increment(x=w179) -> (x+1=w180:i32)
              n59 = GPIB Read(0:w181, 1:w180, 3:w196) -> (5:w188:string, 7:→"Error SR860 Ch1":errorcluster)  [unwired: 2 in, 1 out]
              "Buffer 1" <- w188
              n60 = Unflatten From String(type=sgl[] [], binary string=w188, data includes array or string size? (T)=FALSE, byte order (0:big-endian, network order)=T1."little-endian") -> (value=w184:sgl[])  [unwired: 1 in, 2 out]
              "Buffer 1" <- w184
              n61 = Array Size(array=w184) -> (size(s)=→"size(s) 1":i32)
              n62 = Decimate 1D Array(w184) -> (w183:sgl[], w173:sgl[])
              "R1 Buffer" <- w183
              "T1 Buffer" <- w173
              n63 = call "AC Signal Sign.vi"("Array"=w173) -> ("Sign1"=w172:i8)
              "Sign1" <- w172
              n64 = call <vilib>:"Std Deviation and Variance.vi"("X"=w183) -> ("mean"=w176:dbl, "standard deviation"=w177:dbl)  [unwired: 1 in, 1 out]
              n65 = call <vilib>:"Std Deviation and Variance.vi"("X"=w173) -> ("mean"=w178:dbl, "standard deviation"=w182:dbl)  [unwired: 1 in, 1 out]
              n66 = case shown="True" w174 {
                tunnel: w172 -> [_ w205]
                tunnel: w176 -> [w202 w204]
                tunnel: [w202 w203] -> w175
                frame False {
                }
                frame True {
                  n67 = Multiply(x=w204, y=w205) -> (x*y=w203:dbl)
                }
              }
            }
            frame False {
              w206 = 0.0
            }
          }
        }
      }
      "R1 Mean" <- w116
      "R1 STD" <- w115
      "T1 Mean" <- w114
      "T1 STD" <- w113
    }
  }
